vi "readSettingControls.vi"(8 "error in (no error)":errorcluster, 11 "BaseSetting in":refnum<class "Setting.lvclass">) -> (0 "error out":errorcluster, 3 "BaseSetting out":refnum<class "Setting.lvclass">)   [LabVIEW 2016, in "Settings.lvlib" / "Setting.lvclass"]
uses:
  Setting.lvclass
  Setting.lvclass/Setting.ctl
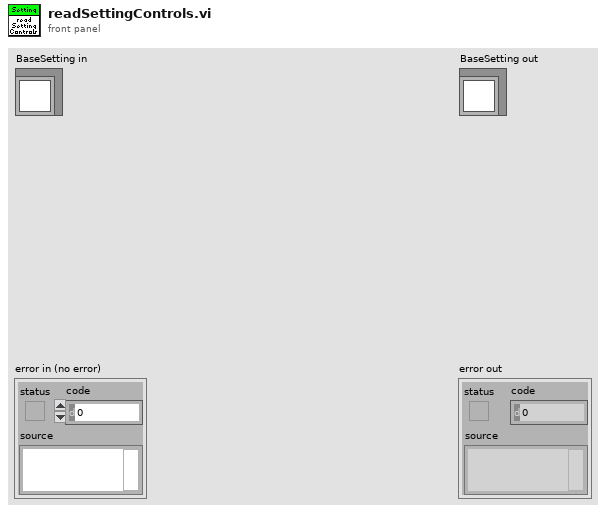
[diagram p1: front panel]
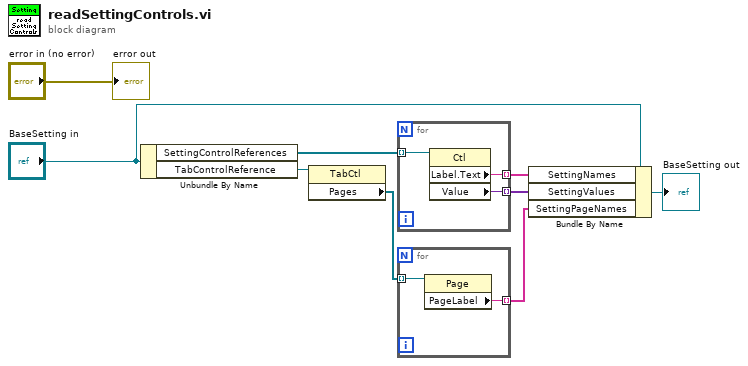
[diagram p0: block diagram]
diagram:
  n1 = Unbundle By Name("BaseSetting in") -> ("SettingControlReferences"=w5:refnum<vi>[], "TabControlReference"=w2:refnum<vi>)
  n2 = property on="Property Node" class="TabCtl"(reference=w2) -> ("Pages"=w3:refnum<vi>[])  [unwired: 1 in, 2 out]
  n3 = for {
    tunnel: w5 -> [w12] mode=indexing
    tunnel: [w11] -> w7 mode=indexing
    tunnel: [w10] -> w6 mode=indexing
    n4 = property class="Ctl"(reference=w12) -> ("Label.Text"=w11:string, "Value"=w10:variant)  [unwired: 1 in, 2 out]
  }
  n5 = for {
    tunnel: w3 -> [w14] mode=indexing
    tunnel: [w13] -> w1 mode=indexing
    n6 = property class="Page"(reference=w14) -> ("PageLabel"=w13:string)  [unwired: 1 in, 2 out]
  }
  n7 = Bundle By Name(cluster="BaseSetting in", "SettingNames"=w7, "SettingValues"=w6, "SettingPageNames"=w1) -> (→"BaseSetting out":refnum<class "Setting.lvclass">)
  "error out" <- "error in (no error)"
